vi "1B_Determine Phase Register.vi"(6 "Address Space Start":u16=125 format="%04x", 7 "Current SEQ":string, 8 "SEQ 1 Stop":string, 9 "SEQ 1 Start":string, 10 "SEQ 0 Stop":string, 11 "SEQ 0 Start":string) -> (1 "Block Read Address Strings":string[](array[string]), 2 "Address Array":u16[](array[numeric]) format="%04x")   [LabVIEW 2010]
panel:
  out "In SEQ 1?":bool
  out "In SEQ 0?":bool
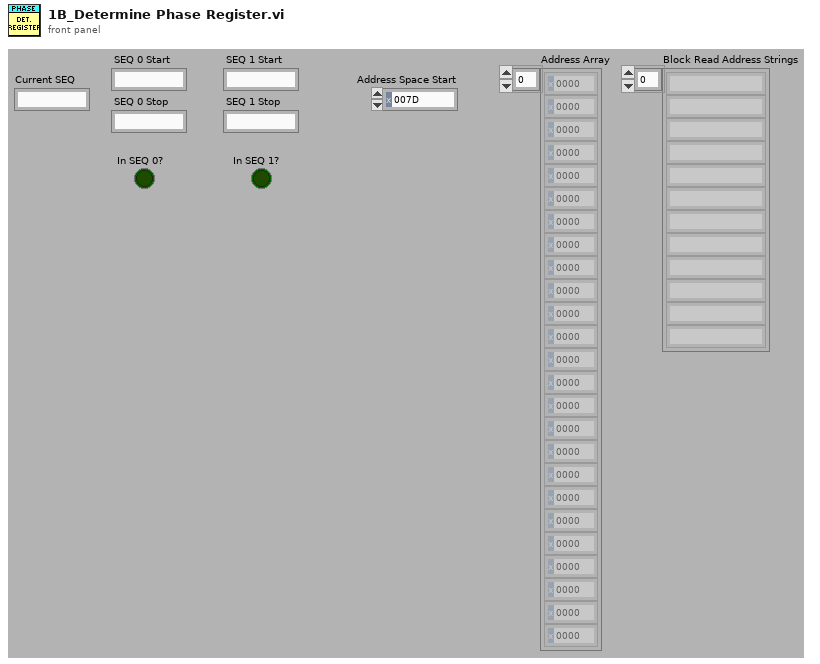
[diagram p1: front panel]
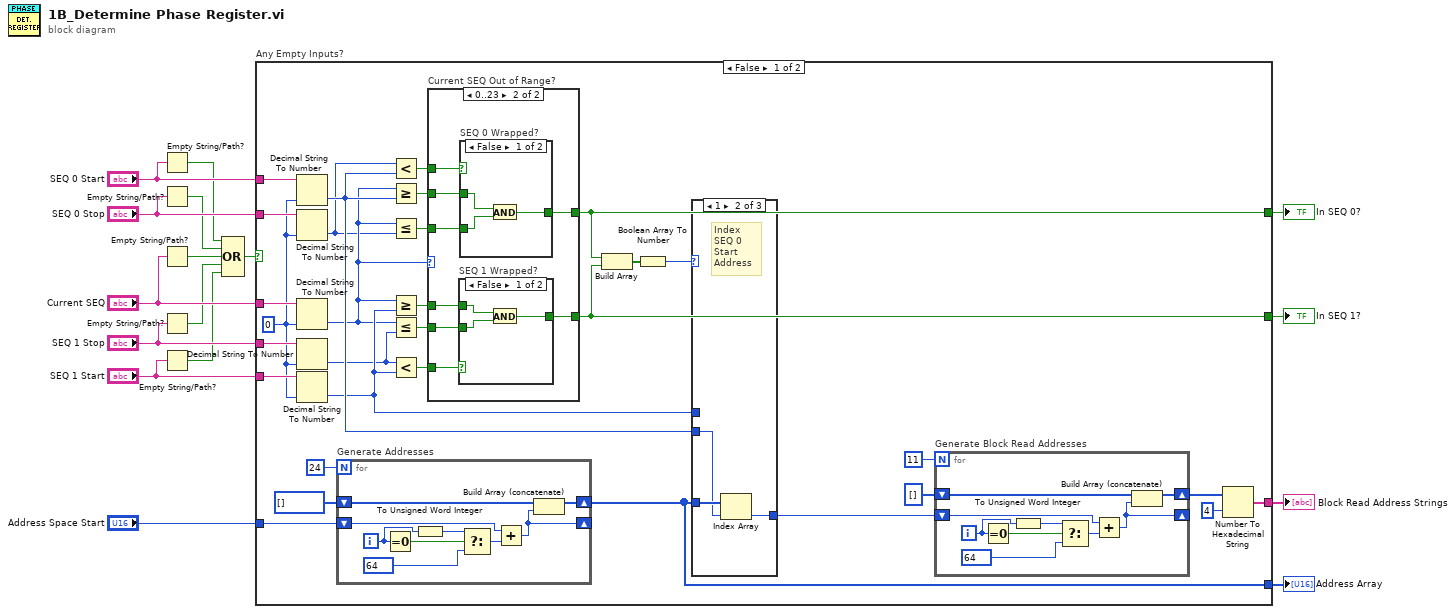
[diagram p0: block diagram]
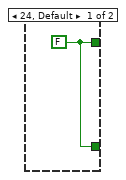
[diagram p2: hidden frame]
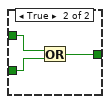
[diagram p3: hidden frame]
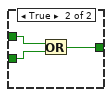
[diagram p4: hidden frame]
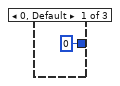
[diagram p5: hidden frame]
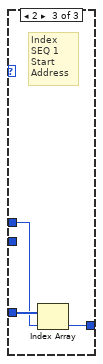
[diagram p6: hidden frame]
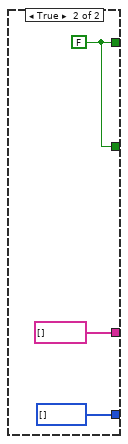
[diagram p7: hidden frame]
diagram:
  n1 = Empty String/Path?(string/path="SEQ 0 Start") -> (empty?=w7:bool)
  n2 = Empty String/Path?(string/path="SEQ 0 Stop") -> (empty?=w8:bool)
  n3 = Empty String/Path?(string/path="Current SEQ") -> (empty?=w9:bool)
  n4 = Empty String/Path?(string/path="SEQ 1 Stop") -> (empty?=w10:bool)
  n5 = Empty String/Path?(string/path="SEQ 1 Start") -> (empty?=w11:bool)
  n6 = Compound Arithmetic op=OR(w7, w8, w9, w10, w11) -> (w1:bool)
  n7 = case "Any Empty Inputs?" shown="False" w1 {
    tunnel: "SEQ 1 Stop" -> [w47 _]
    tunnel: "SEQ 1 Start" -> [w46 _]
    tunnel: "Current SEQ" -> [w45 _]
    tunnel: "SEQ 0 Stop" -> [w44 _]
    tunnel: "SEQ 0 Start" -> [w43 _]
    tunnel: "Address Space Start" -> [w42 _]
    tunnel: [w41 w94] -> w5
    tunnel: [w40 w94] -> w4
    tunnel: [w32 u16[] []] -> w3
    tunnel: [w29 string[] []] -> w2
    frame False {
      w28 = u8 0 ("default (0 I32)")
      n8 = Decimal String To Number(string=w43, default (0L)=w28) -> (number=w37:u8)  [unwired: 1 in, 1 out]
      n9 = Decimal String To Number(string=w44, default (0L)=w28) -> (number=w18:u8)  [unwired: 1 in, 1 out]
      n10 = Decimal String To Number(string=w45, default (0L)=w28) -> (number=w19:u8)  [unwired: 1 in, 1 out]
      n11 = Decimal String To Number(string=w47, default (0L)=w28) -> (number=w17:u8)  [unwired: 1 in, 1 out]
      n12 = Decimal String To Number(string=w46, default (0L)=w28) -> (number=w36:u8)  [unwired: 1 in, 1 out]
      n13 = for "Generate Addresses" {
        N: 24 -> [_]
        shift-right: [w55] -> _
        shift-left: w42 -> [w56]
        shift-right: [w54] -> w32
        shift-left: u16[] [] -> [w53]
        i -> [w51]
        n14 = Equal To 0?(x=w51) -> (x = 0?=w50:bool)
        n15 = To Unsigned Word Integer(number=w51) -> (unsigned 16bit integer=w48:u16)
        n16 = Select(t=w48, s=w50, f=u16 64 ("Start Address")) -> (s? t:f=w49:u16)
        n17 = Add(x=w56, y=w49) -> (x+y=w55:u16)
        n18 = Build Array (concatenate)(w53, w55) -> (w54:u16[])
      }
      n19 = Less?(x=w18, y=w37) -> (x < y?=w22:bool)
      n20 = Greater Or Equal?(x=w19, y=w37) -> (x >= y?=w24:bool)
      n21 = Less Or Equal?(x=w19, y=w18) -> (x <= y?=w23:bool)
      n22 = Greater Or Equal?(x=w19, y=w36) -> (x >= y?=w26:bool)
      n23 = Less Or Equal?(x=w19, y=w17) -> (x <= y?=w27:bool)
      n24 = Less?(x=w17, y=w36) -> (x < y?=w25:bool)
      n25 = case "Current SEQ Out of Range?" shown="0..23" w19 {
        tunnel: w27 -> [_ w65]
        tunnel: w26 -> [_ w64]
        tunnel: [w57 w63] -> w40
        tunnel: w25 -> [_ w62]
        tunnel: w24 -> [_ w61]
        tunnel: w23 -> [_ w60]
        tunnel: w22 -> [_ w59]
        tunnel: [w57 w58] -> w41
        frame 24, Default {
          w57 = FALSE
        }
        frame 0..23 {
          n26 = case "SEQ 1 Wrapped?" shown="False" w62 {
            tunnel: w65 -> [w74 w75]
            tunnel: w64 -> [w73 w76]
            tunnel: [w72 w77] -> w63
            frame False {
              n27 = And(x=w73, y=w74) -> (x .and. y?=w72:bool)
            }
            frame True {
              n28 = Or(x=w76, y=w75) -> (x .or. y?=w77:bool)
            }
          }
          n29 = case "SEQ 0 Wrapped?" shown="False" w59 {
            tunnel: w60 -> [w68 w69]
            tunnel: w61 -> [w67 w70]
            tunnel: [w66 w71] -> w58
            frame False {
              n30 = And(x=w67, y=w68) -> (x .and. y?=w66:bool)
            }
            frame True {
              n31 = Or(x=w70, y=w69) -> (x .or. y?=w71:bool)
            }
          }
        }
      }
      n32 = Build Array(w41, w40) -> (w39:bool[])
      n33 = Boolean Array To Number(Boolean array=w39) -> (number=w38:u32)
      n34 = case shown="1" w38 {
        tunnel: w32 -> [_ w89 w93]
        tunnel: w37 -> [_ w88 _]
        tunnel: w36 -> [_ _ w91]
        tunnel: [u16 0 w90 w92] -> w33
        frame 0, Default {
        }
        frame 1 {
          # "Index\nSEQ 0\nStart\nAddress"
          n35 = Index Array(array=w89, index=w88) -> (element=w90:u16)
        }
        frame 2 {
          # "Index\nSEQ 1\nStart\nAddress"
          n36 = Index Array(array=w93, index=w91) -> (element=w92:u16)
        }
      }
      n37 = for "Generate Block Read Addresses" {
        N: 11 -> [_]
        shift-right: [w85] -> _
        shift-left: w33 -> [w86]
        shift-right: [w84] -> w31
        shift-left: u16[] [] -> [w83]
        i -> [w81]
        n38 = Equal To 0?(x=w81) -> (x = 0?=w80:bool)
        n39 = To Unsigned Word Integer(number=w81) -> (unsigned 16bit integer=w78:u16)
        n40 = Select(t=w78, s=w80, f=u16 64 ("Start Address")) -> (s? t:f=w79:u16)
        n41 = Add(x=w86, y=w79) -> (x+y=w85:u16)
        n42 = Build Array (concatenate)(w83, w85) -> (w84:u16[])
      }
      n43 = Number To Hexadecimal String(1:i16 4 ("width (-)"), 2:w31) -> (0:w29:string[])
    }
    frame True {
      w94 = FALSE
    }
  }
  "In SEQ 0?" <- w5
  "In SEQ 1?" <- w4
  "Address Array" <- w3
  "Block Read Address Strings" <- w2
